vi "ErrorMSG_error&warning situation control.vi"(1 "error&warning control":T1(ring)) -> ()   [LabVIEW 2019]
doc: "By error&warning control selection,it reflects different situation control of tripple light tower & button light,see code inside to comprehend define of those situation"
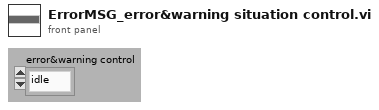
[diagram p1: front panel]
types:
  T1 = enum16{"idle", "error occurs", "warning occurs", "error cleared", "warning cleared", "run"}
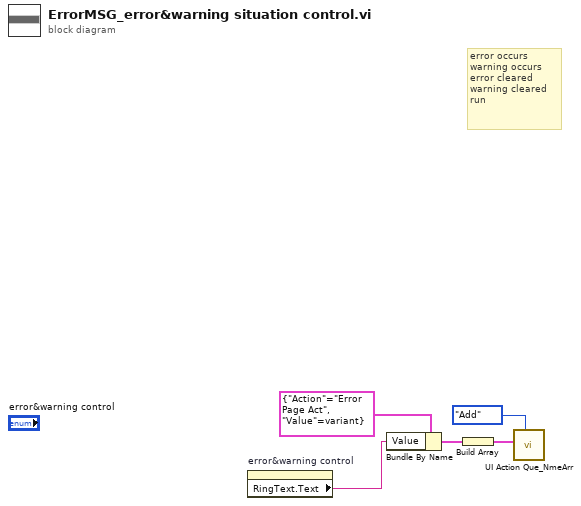
[diagram p0: block diagram]
diagram:
  # "error occurs\nwarning occurs\nerror cleared\nwarning cleared\nrun"
  n1 = property on="error&warning control" class="Enum (strict)"() -> ("RingText.Text"=w1:string)  [unwired: 2 in, 2 out]
  n2 = Bundle By Name(cluster=cluster{"Action":string, "Value":variant} {"Action"="Error Page Act", "Value"=variant} ("UI Action"), "Value"=w1) -> (w3:cluster{"Action":string, "Value":variant})
  n3 = Build Array(w3) -> (w2:cluster{"Action":string, "Value":variant}[])
  n4 = call "UI Action Que_NmeArr.vi"("Action"=enum16{"Initial", "Add", "Release"}."Add", "UI Process"=w2) -> ()  [unwired: 8 in, 2 out]
